vi "LowerStop_example.vi"   [LabVIEW 2016]
uses:
  Classes/Controller/Controller Folder/Controller.lvclass
types:
  T1 = typedef "Controller.lvclass/Controllers.ctl" = cluster{"Copy of Motion.lvclass":refnum<class "Motion.lvclass">, "Copy of I-O.lvclass ":refnum<class "I-O.lvclass">, "Copy of Dispenser.lvclass":refnum<class "Dispenser.lvclass">}
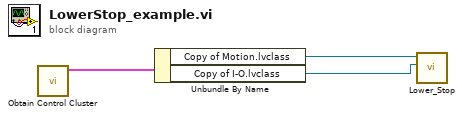
[diagram p0: block diagram]
diagram:
  n1 = call "Obtain Control Cluster.vi"() -> ("Control Out"=w3:T1)  [unwired: 11 in]
  n2 = Unbundle By Name(w3) -> ("Copy of Motion.lvclass"=w2:refnum<class "Motion.lvclass">, "Copy of I-O.lvclass"=w1:refnum<class "I-O.lvclass">)
  n3 = call "Lower_Stop.vi"("I-O in"=w1, "Motion in"=w2) -> ()  [unwired: 7 in, 3 out]
